vi "220326_STEPN_OCR_v12.vi"(5 "Mode":enum16{"walking", "Repair", "wallet Balance"}(ring), 6 "path to PNG file":path=path "G:/マイドライブ/STEPN_walking/PNG/IMG_5909.PNG" caption="PNG single path") -> (0 "item":string[](array[string])=["Run time", "Step", "Earn GST", "Energy", "Distance", "Date time", "Shoe Lv.", "Shoe #", "durability", "-repair"], 1 "Output String":string[](array[string]), 2 "reading path":path=path "G:/マイドライブ/STEPN_walking/IMG_5909.PNG" caption="PNG single path", 3 "elapsed time(s)":dbl[][](array[numeric]) format="%#_3g", 4 "moji N":i32[](array[numeric]))   [LabVIEW 2016]
uses:
  <vilib>/Utility/file.llb/Write Delimited Spreadsheet (string).vi
  <vilib>/picture/picture.llb/imagedata.ctl
panel:
  out "Boolean":bool
  out "Sumtime(s)":dbl
  in  "File save":bool
  in  "タブ制御器":T1(tab)
  in  "Repair":T2(array[cluster])=[{"left"=300, "top"=529, "right"=508, "bottom"=569}, {"left"=300, "top"=648, "right"=560, "bottom"=677}, {"left"=356, "top"=697, "right"=460, "bottom"=742}]
  in  "walking range":T2(array[cluster])=[{"left"=30, "top"=439, "right"=620, "bottom"=479}, {"left"=430, "top"=668, "right"=620, "bottom"=708}, {"left"=440, "top"=762, "right"=620, "bottom"=802}, {"left"=378, "top"=248, "right"=565, "bottom"=300}, {"left"=123, "top"=296, "right"=350, "bottom"=316}, {"left"=100, "top"=644, "right"=290, "bottom"=664}, {"left"=160, "top"=845, "right"=279, "bottom"=865}, {"left"=150, "top"=891, "right"=242, "bottom"=907}, {"left"=290, "top"=891, "right"=328, "bottom"=907}] caption="walking"
  out "Input picture":picture caption="新規ピクチャ"
  out "image data":T3 caption="画像データ"
  in  "Wallet Balance":T2(array[cluster])=[{"left"=300, "top"=770, "right"=591, "bottom"=830}, {"left"=300, "top"=870, "right"=591, "bottom"=930}, {"left"=300, "top"=970, "right"=591, "bottom"=1030}, {"left"=300, "top"=1070, "right"=591, "bottom"=1130}] caption="wallet Balance"
  out "RANGE":picture
  out "Array":i32[][](array[numeric])
  in  "new flame":T2(array[cluster])=[{"left"=30, "top"=439, "right"=620, "bottom"=479}, {"left"=430, "top"=668, "right"=620, "bottom"=708}, {"left"=440, "top"=762, "right"=620, "bottom"=802}, {"left"=378, "top"=248, "right"=565, "bottom"=300}, {"left"=123, "top"=296, "right"=350, "bottom"=316}, {"left"=100, "top"=644, "right"=290, "bottom"=664}, {"left"=160, "top"=845, "right"=279, "bottom"=865}, {"left"=150, "top"=891, "right"=242, "bottom"=907}, {"left"=290, "top"=891, "right"=328, "bottom"=907}] caption="NEW RANGE"
  in  "RANGE No.":i32
  in  "Range search 2":bool
  out "4-bit pixmap":u8[][][][](array[numeric])
  out "Resized pixmap 2":u8[][][](array[numeric])
  out "string N":i32[](array[numeric])
  in  "new file path (Not A Path if cancelled)":path=path "G:/マイドライブ/STEPN_csv" caption="Save to Path"
  out "Save filename":path
  out "Resized N1 pixmap":i32[][](array[numeric])
  out "N1 Input pic.":picture caption="N1test pic."
  in  "picture No.":i32[](array[numeric])
  out "testdata":T3
  out "identify %":dbl[](array[numeric])
  out "max identify %":dbl
  out "OCR Number":i32
  out "pixcel size (V, Y)":i32[](array[numeric])
  out "Resized (Y, X)":i32[](array[numeric])
  out "Output string":string
  out "Resized N1 pic.":picture caption="Output pic."
  out "Input N1 (Y, X)":i32[](array[numeric])
  out "Ref. pic.":picture caption="fixed pic."
  out "pixcel size(X,Y)":i32[][](array[numeric])
  out "OUtput OCR":string[](array[string])
  out "snipper elapsed time(s) 2":dbl[][][](array[numeric]) format="%.2g"
  out "String":string[](array[string])
  in  "N1_test":bool
  in  "Range search":bool
  out "insert_N":i32[](array[numeric])
  out "max identify % 2":dbl[](array[numeric]) format="%#_3g"
  out "cut picture":picture[](array[picture])
  out "pixel size before":i32[][](array[numeric])
  out "OUtput OCR 2":string[](array[string])
  out "Resized (Y,X)":i32[][](array[numeric])
  out "Resized pic.":picture[](array[picture])
  # "LIST\n0 : runT, STEP (40×30)\n1 : Earn GST (40×30)\n2 : Energy (40×30)\n3 : distance (52×39)\n4 : Date time (20×15)\n5 : shoe Lv. (20×15)\n6 : shoe # (20×15)\n7 : durability (16×12)\n8 : -repair (16×12)"
  # "second"
  # "second"
  # "%"
  # "1"
  # "2"
  # "3"
  # "4"
  # "5"
  # "6"
  # "OFF"
  # "ON"
  # "OFF"
  # "ON"
  # "画像塊"
  # "番号"
  # "OFF"
  # "ON"
  # "c15~¡"
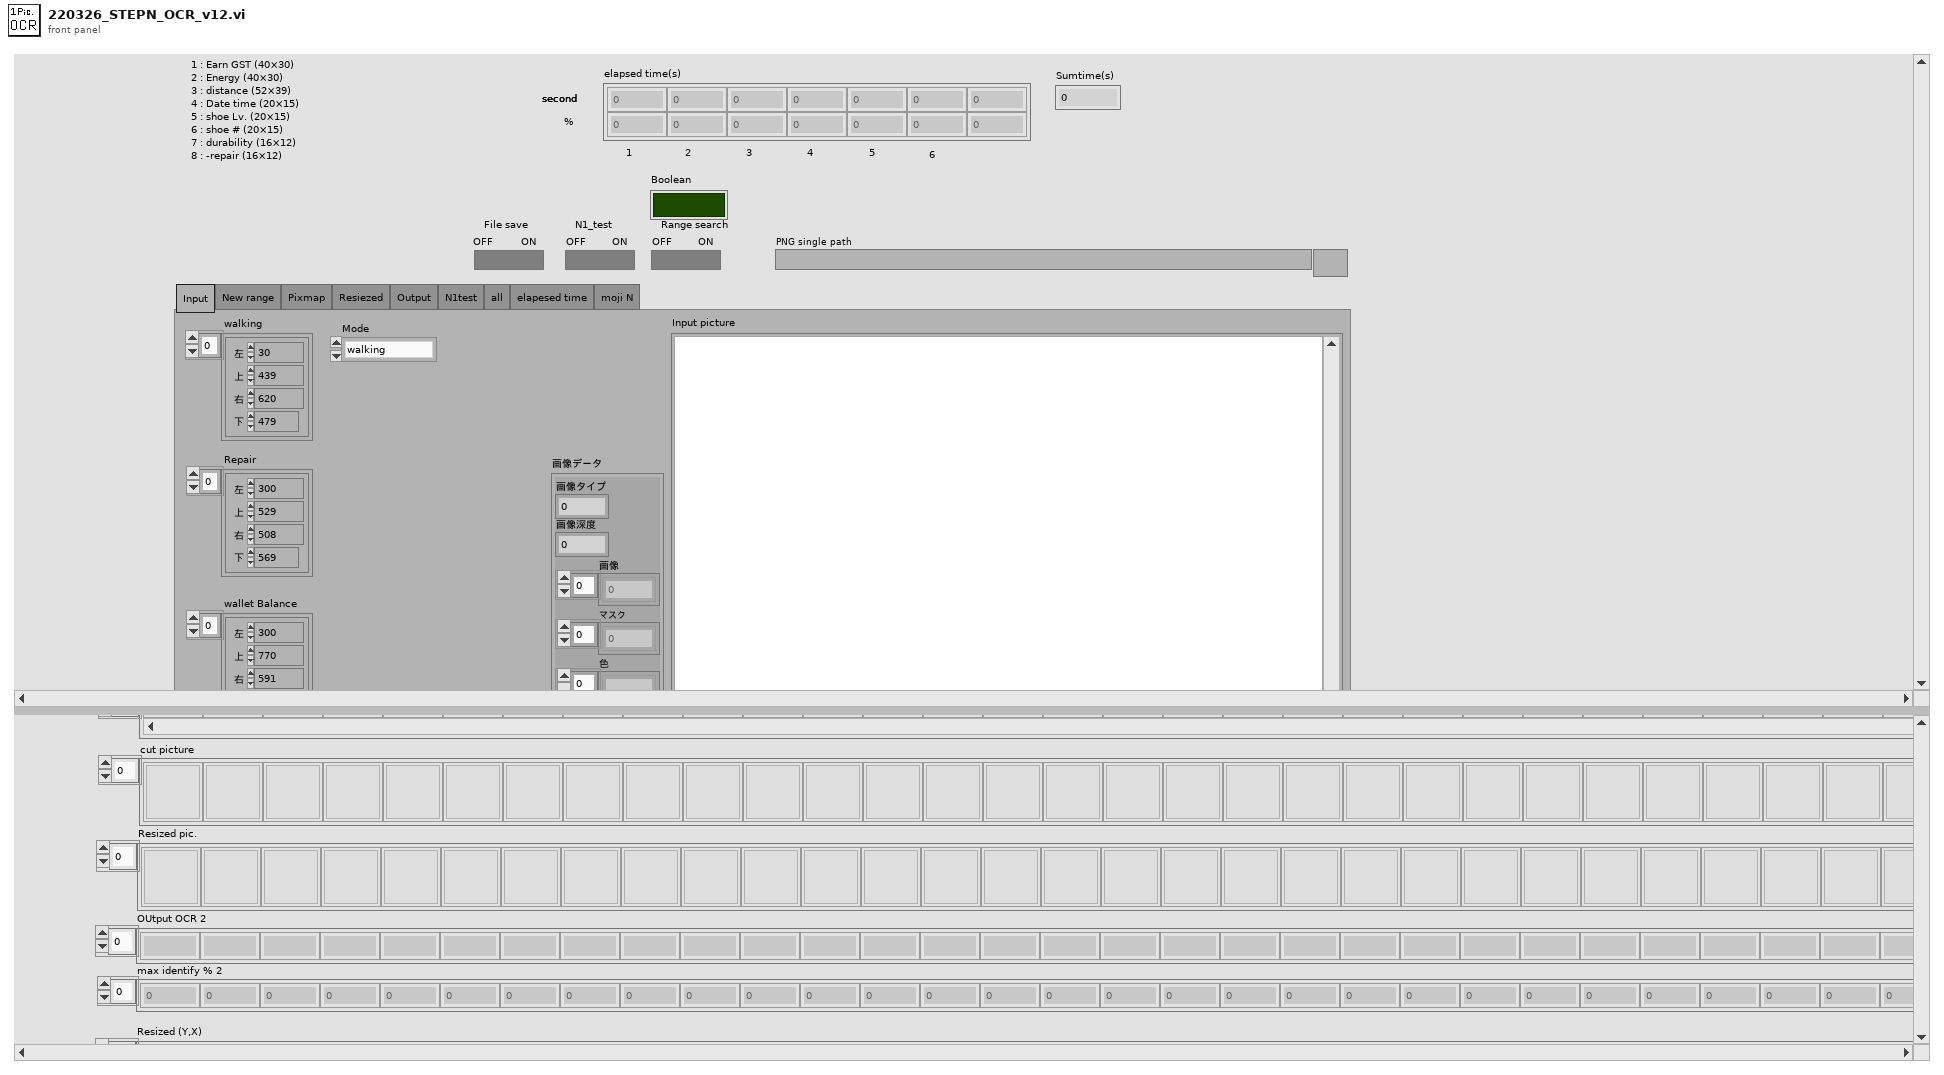
[diagram p1: front panel]
types:
  T1 = enum32{"Input", "New range", "Pixmap", "Resiezed", "Output", "N1test", "all", "elapesed time", "moji N"}
  T2 = cluster{"left":i16, "top":i16, "right":i16, "bottom":i16}[]
  T3 = typedef "imagedata.ctl" = cluster{"image type":i32, "image depth":i32, "image":u8[], "mask":u8[], "colors":u32[], "Rectangle":cluster{"left":i16, "top":i16, "right":i16, "bottom":i16}}
  T4 = cluster{"left":i16, "top":i16, "right":i16, "bottom":i16}
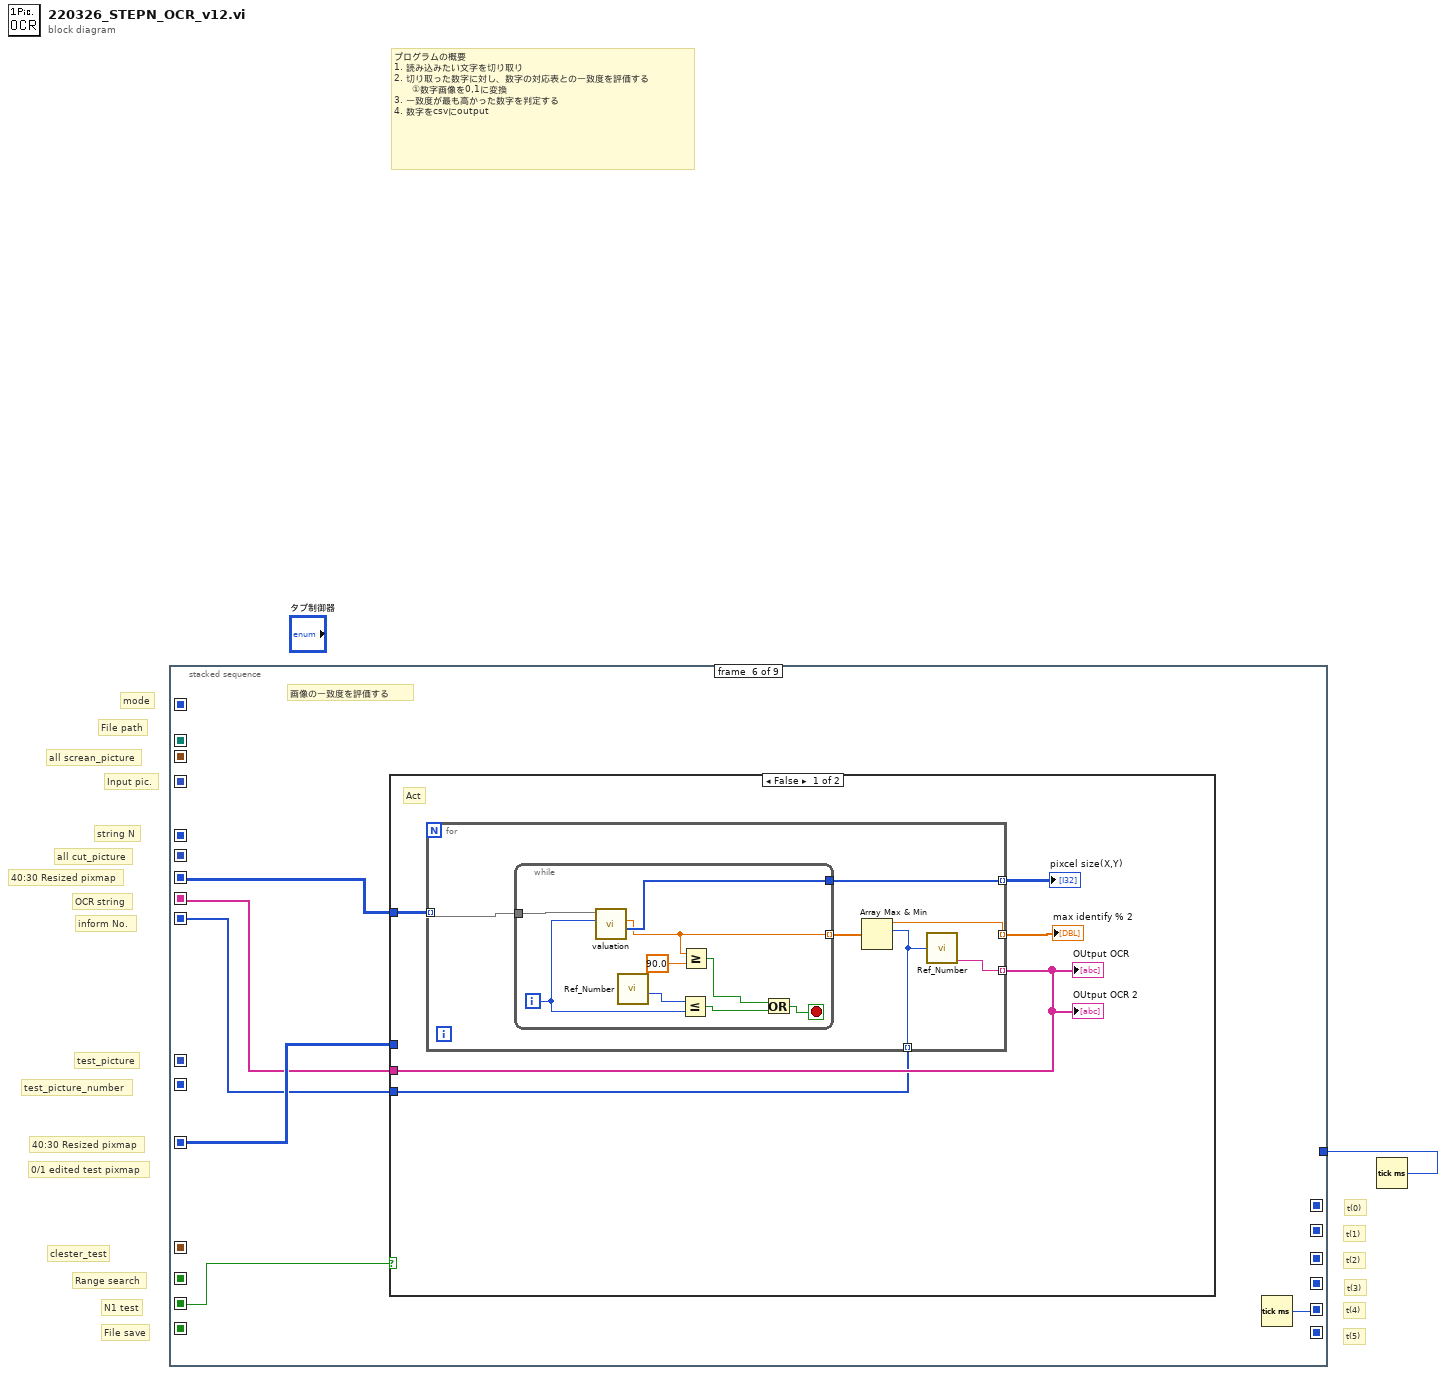
[diagram p0: block diagram]
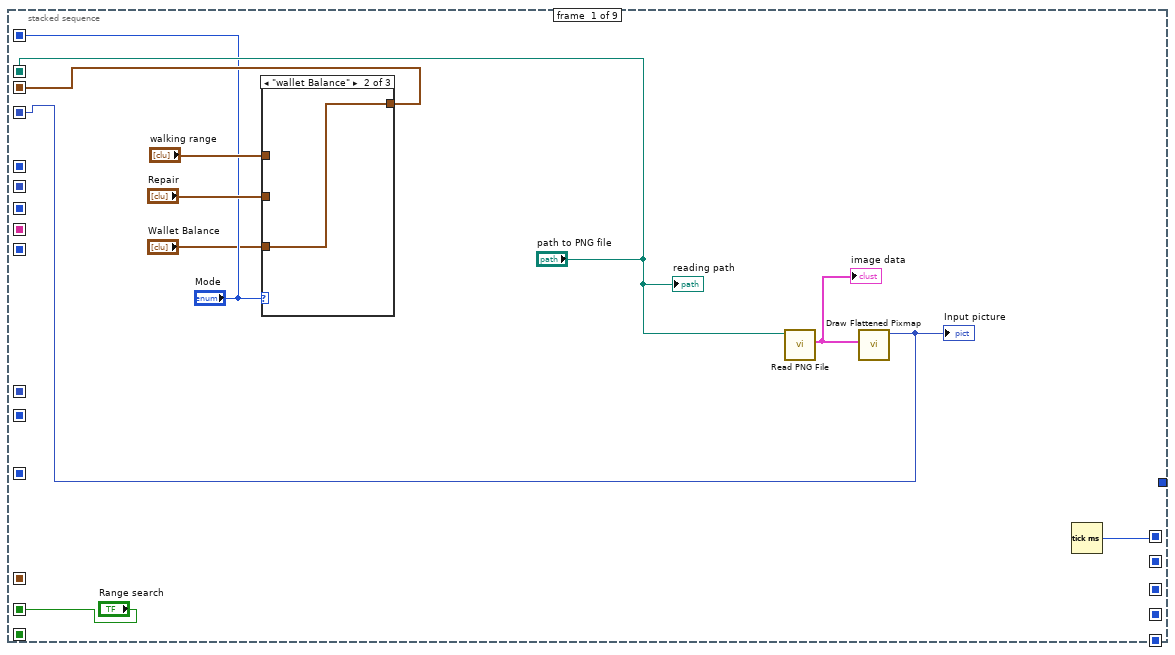
[diagram p2: hidden frame]
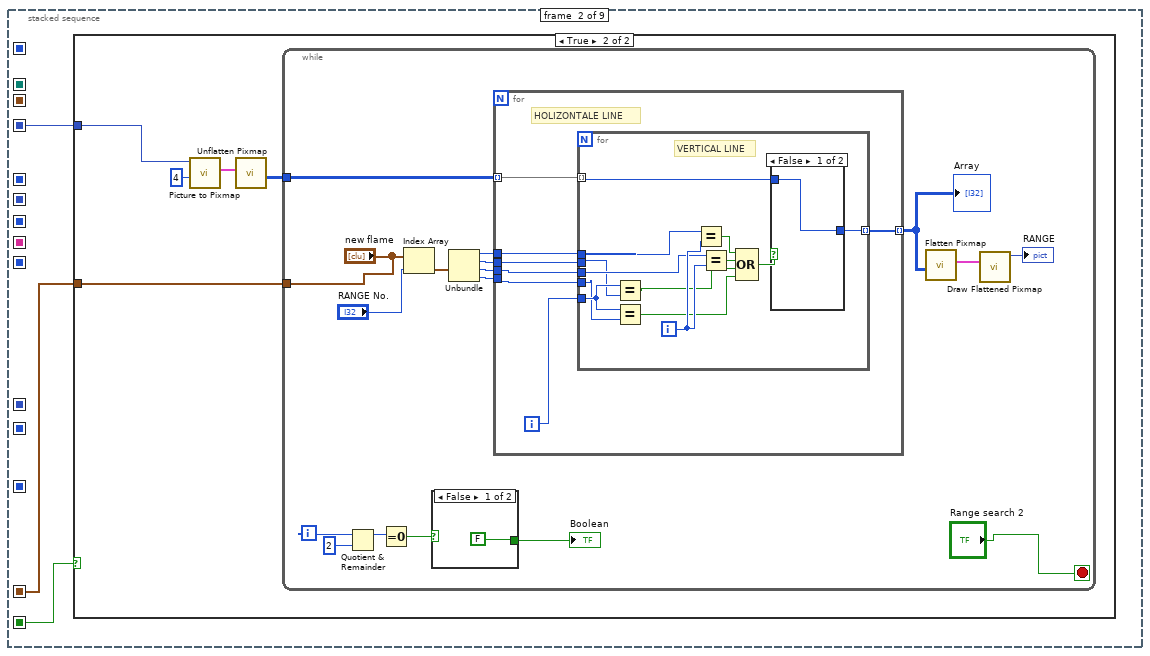
[diagram p5: hidden frame]
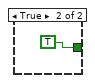
[diagram p7: hidden frame]
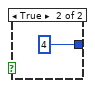
[diagram p8: hidden frame]
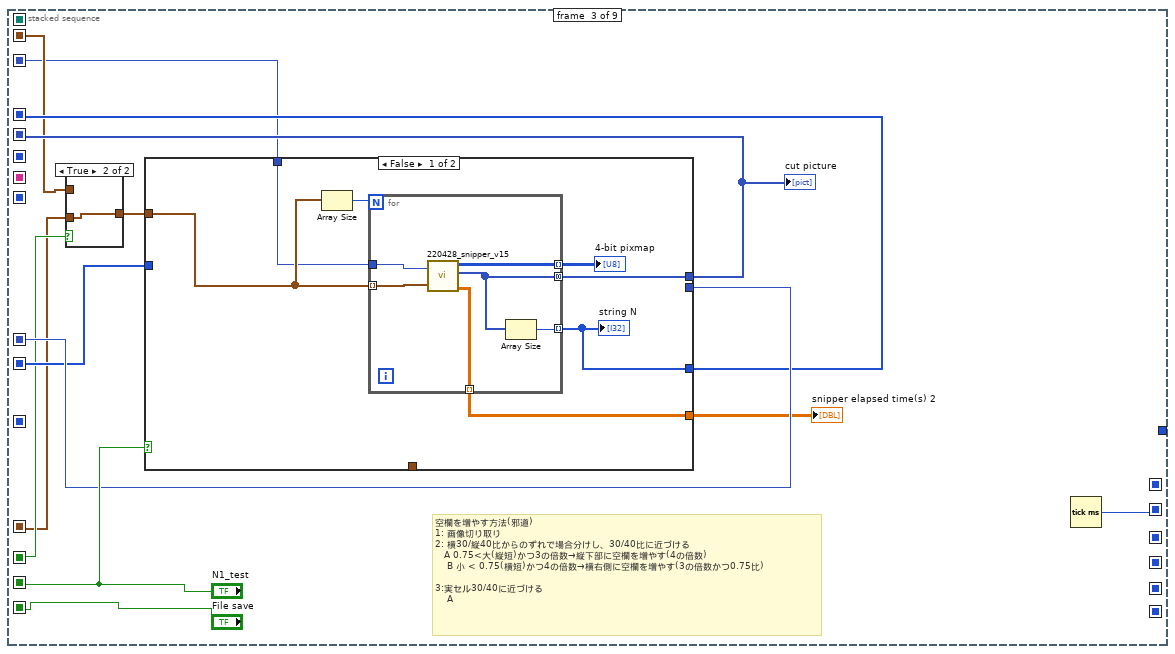
[diagram p9: hidden frame]
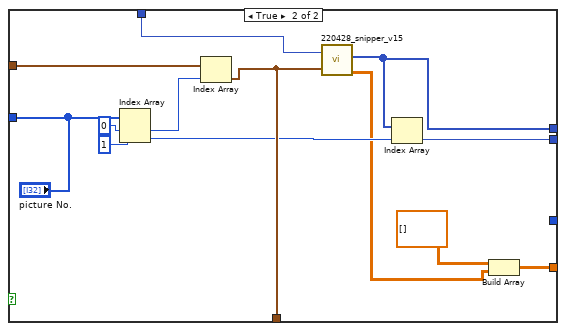
[diagram p11: hidden frame]
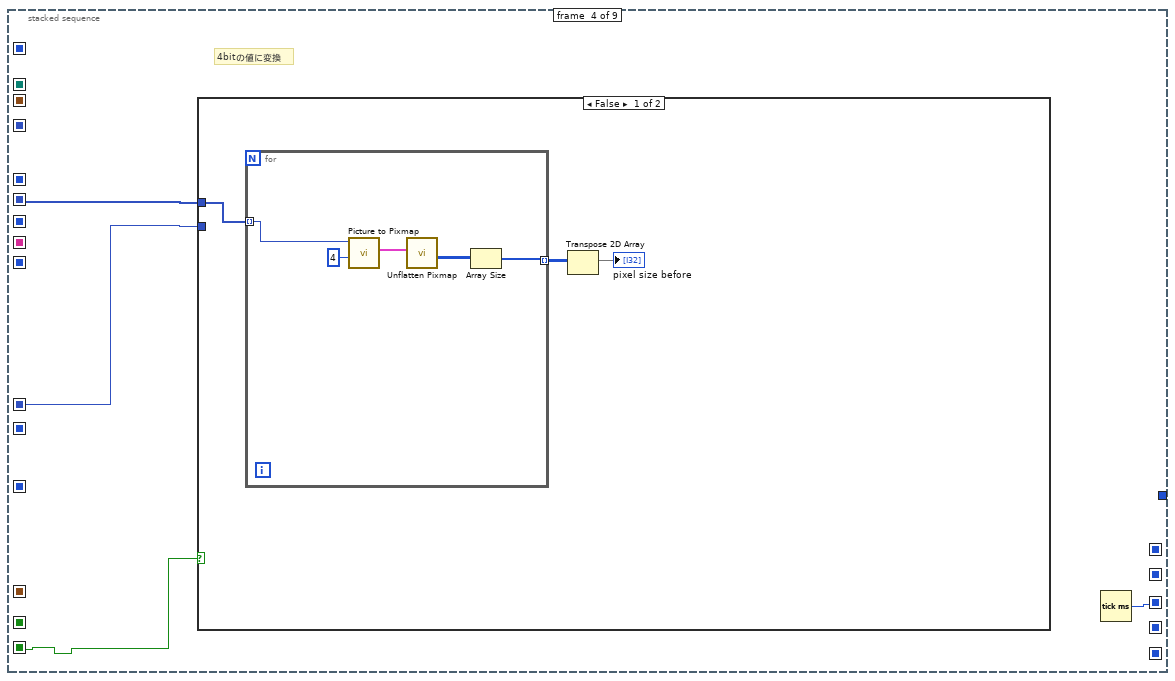
[diagram p12: hidden frame]
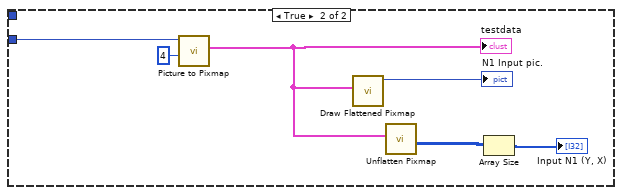
[diagram p13: hidden frame]
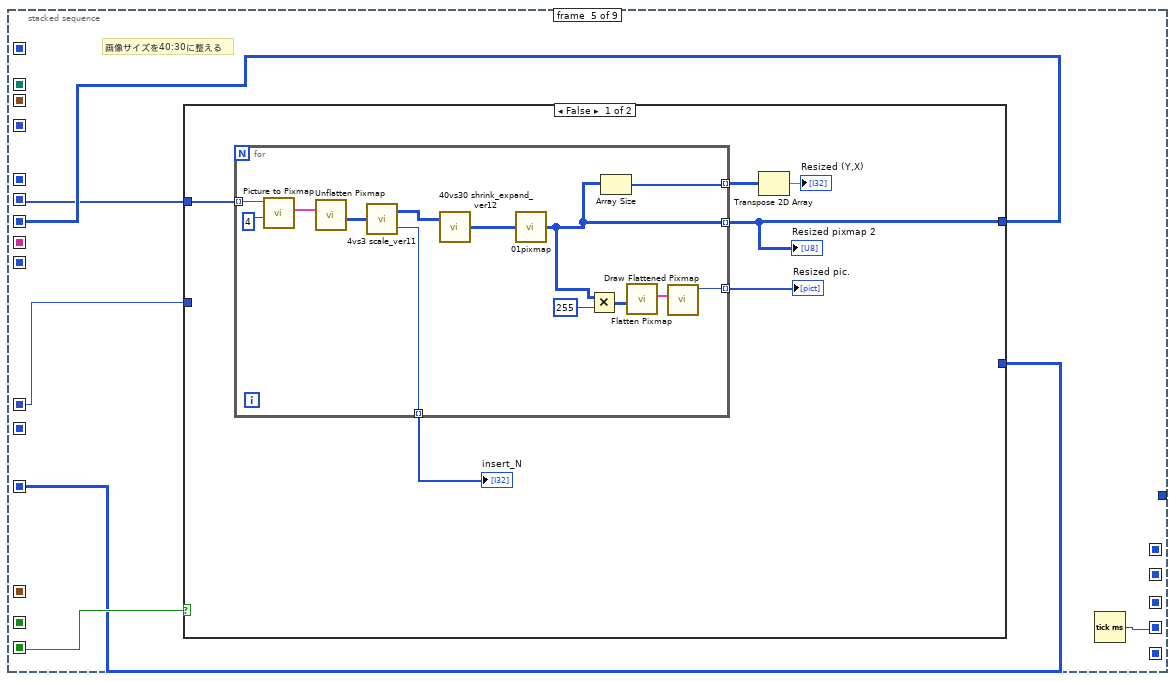
[diagram p14: hidden frame]
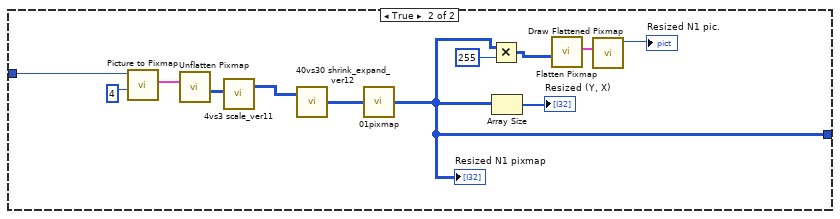
[diagram p15: hidden frame]
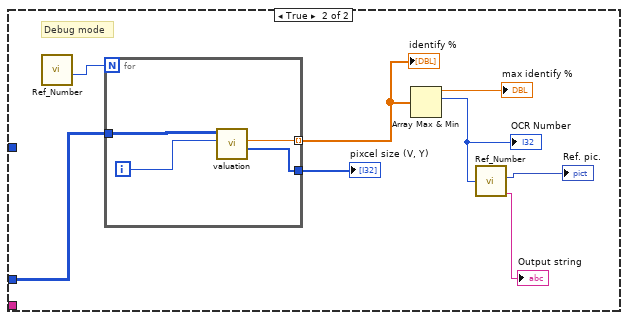
[diagram p16: hidden frame]
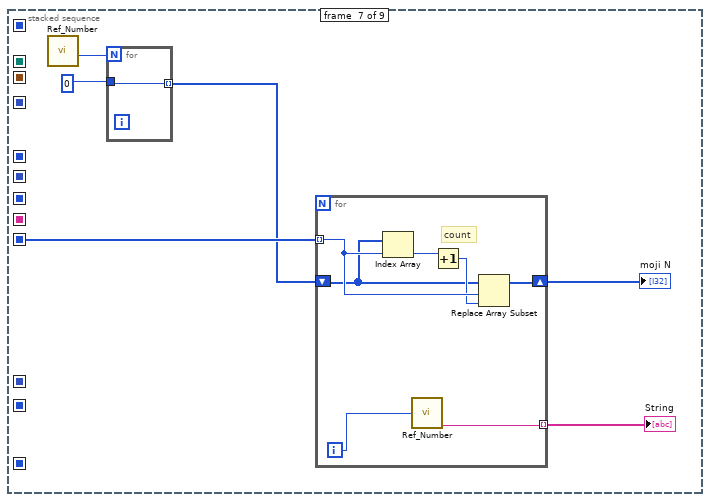
[diagram p17: hidden frame]
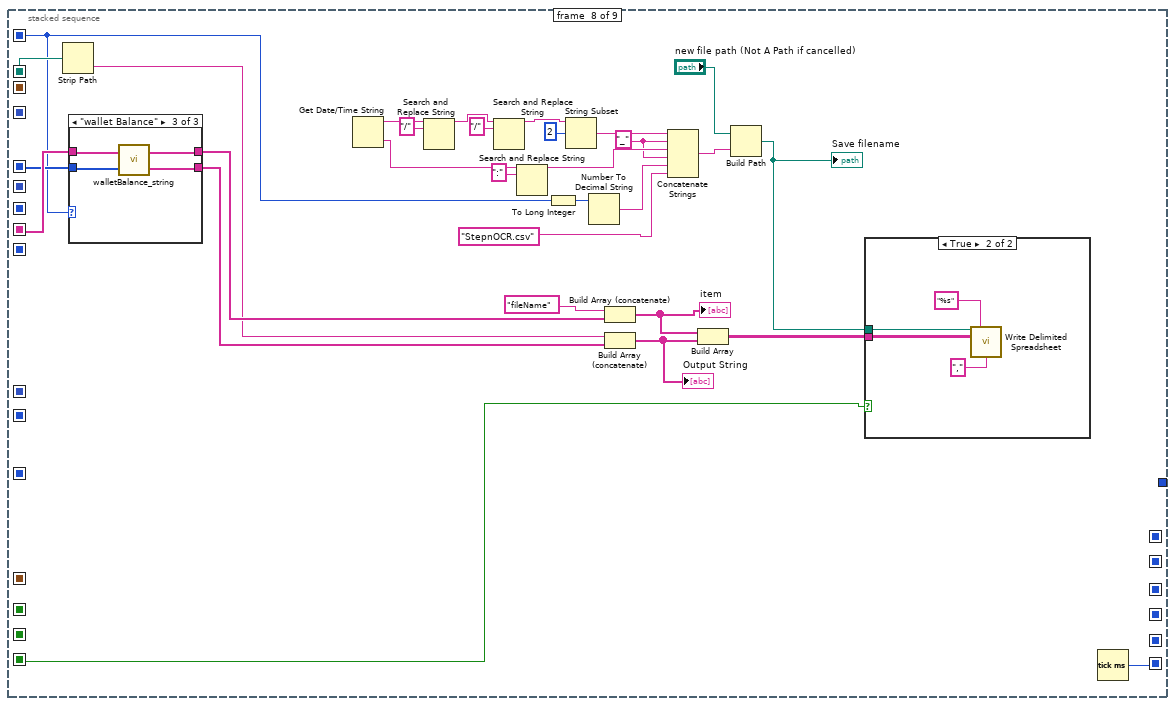
[diagram p18: hidden frame]
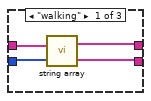
[diagram p19: hidden frame]
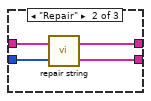
[diagram p20: hidden frame]
diagram:
  # "Input pic."
  # "mode"
  # "inform No."
  # "t(5)"
  # "t(4)"
  # "t(3)"
  # "t(2)"
  # "t(1)"
  # "t(0)"
  # "File save"
  # "string N"
  # "OCR string"
  # "40:30 Resized pixmap"
  # "40:30 Resized pixmap"
  # "0/1 edited test pixmap"
  # "all screan_picture"
  # "all cut_picture"
  # "File path"
  # "clester_test"
  # "test_picture_number"
  # "test_picture"
  # "Range search"
  # "N1 test"
  # "プログラムの概要\n1. 読み込みたい文字を切り取り\n2. 切り取った数字に対し、数字の対応表との一致度を評価する\n　　①数字画像を0,1に変換\n3. 一致度が最も高かった数字を判定する\n4. 数字をcsvにoutput"
  n1 = Tick Count (ms)() -> (millisecond timer value=w1:u32)
  n2 = stacked-sequence {
    seq-local: [_ _ "N1_test" _ _ _ _ _ _] -> [_ _ _ w108 w128 w165 _ _ _]
    seq-local: [_ w16 _ _ _ _ _ _ _] -> [_ _ w65 _ _ _ _ _ _]
    seq-local: ["path to PNG file" _ _ _ _ _ _ _ _] -> [_ _ _ _ _ _ _ w223 _]
    seq-local: [_ _ w75 _ _ _ _ _ _] -> [_ _ _ w106 w124 _ _ _ _]
    seq-local: [_ _ w73 _ _ _ _ _ _] -> [_ _ _ w107 w126 _ _ _ _]
    seq-local: [_ _ w74 _ _ _ _ _ _] -> [_ _ _ _ _ _ _ _ _]
    seq-local: ["Range search" _ _ _ _ _ _ _ _] -> [_ w17 w66 _ _ _ _ _ _]
    seq-local: [_ _ _ _ w125 _ _ _ _] -> [_ _ _ _ _ w163 _ _ _]
    seq-local: [_ _ _ _ w127 _ _ _ _] -> [_ _ _ _ _ w164 _ _ _]
    seq-local: [_ _ _ _ _ w162 _ _ _] -> [_ _ _ _ _ _ _ w241 _]
    seq-local: [_ _ w72 _ _ _ _ _ _] -> [_ _ _ _ _ _ _ w240 _]
    seq-local: [_ _ "File save" _ _ _ _ _ _] -> [_ _ _ _ _ _ _ w224 _]
    seq-local: [w9 _ _ _ _ _ _ _ _] -> [_ _ _ _ _ _ _ _ w269]
    seq-local: [_ _ w70 _ _ _ _ _ _] -> [_ _ _ _ _ _ _ _ w268]
    seq-local: [_ _ _ w105 _ _ _ _ _] -> [_ _ _ _ _ _ _ _ w267]
    seq-local: [_ _ _ _ w123 _ _ _ _] -> [_ _ _ _ _ _ _ _ w266]
    seq-local: [_ _ _ _ _ w161 _ _ _] -> [_ _ _ _ _ _ _ _ w265]
    seq-local: [_ _ _ _ _ _ _ w216 _] -> [_ _ _ _ _ _ _ _ w264]
    seq-local: [_ _ _ _ _ w160 _ _ _] -> [_ _ _ _ _ _ w203 _ _]
    seq-local: [w5 _ _ _ _ _ _ _ _] -> [_ _ w67 _ _ _ _ _ _]
    seq-local: ["Mode" _ _ _ _ _ _ _ _] -> [_ _ _ _ _ _ _ w212 _]
    seq-local: [w2 _ _ _ _ _ _ _ _] -> [_ w15 w64 _ _ _ _ _ _]
    tunnel: w1 -> [_ _ _ _ _ _ _ _ w263]
    frame #0 {
      n3 = case shown="\"wallet Balance\"" "Mode" {
        tunnel: "Repair" -> [w12 _ _]
        tunnel: "walking range" -> [_ _ w14]
        tunnel: [w12 w13 w14] -> w5
        tunnel: "Wallet Balance" -> [_ w13 _]
        frame "Repair" {
        }
        frame "wallet Balance" {
        }
        frame "walking" {
        }
      }
      n4 = call <vilib>:"Read PNG File.vi"("path to PNG file"="path to PNG file") -> ("image data"=w11:T3)  [unwired: 8 in, 2 out]
      "image data" <- w11
      n5 = call <vilib>:"Draw Flattened Pixmap.vi"("image data"=w11) -> ("new picture"=w2:picture)  [unwired: 8 in]
      "Input picture" <- w2
      n6 = Tick Count (ms)() -> (millisecond timer value=w9:u32)
      "reading path" <- "path to PNG file"
    }
    frame #1 {
      n7 = case shown="True" w17 {
        tunnel: [_ w22] -> w16
        tunnel: w15 -> [_ w18]
        frame False {
        }
        frame True {
          n8 = call <vilib>:"Picture to Pixmap.vi"("depth"=4, "picture"=w18) -> ("image data"=w21:T3)  [unwired: 8 in, 1 out]
          n9 = call <vilib>:"Unflatten Pixmap.vi"("image data"=w21) -> ("4-bit pixmap"=w19:u8[][])  [unwired: 4 in, 6 out]
          n10 = while {
            tunnel: w19 -> [w37]
            tunnel: ["new flame"] -> w22
            i -> [w27]
            stop <- "Range search 2" stop-if-true
            n11 = Quotient & Remainder(x=w27, y=2) -> (x-y*floor(x/y)=w25:i32)  [unwired: 1 out]
            n12 = Equal To 0?(x=w25) -> (x = 0?=w24:bool)
            n13 = Index Array(array="new flame", index="RANGE No.") -> (element=w38:T4)
            n14 = case shown="False" w24 {
              tunnel: [FALSE TRUE] -> w23
              frame False {
              }
              frame True {
              }
            }
            "Boolean" <- w23
            n15 = Unbundle(w38) -> ("left"=w31:i16, "top"=w36:i16, "right"=w30:i16, "bottom"=w35:i16)
            n16 = for {
              tunnel: w37 -> [w48] mode=indexing
              tunnel: [w47] -> w34 mode=indexing
              tunnel: w36 -> [w46]
              tunnel: w35 -> [w42]
              tunnel: w31 -> [w45]
              tunnel: w30 -> [w44]
              i -> [w43]
              # "HOLIZONTALE LINE"
              n17 = for {
                tunnel: w48 -> [w58] mode=indexing
                tunnel: [w61] -> w47 mode=indexing
                tunnel: w46 -> [w54]
                tunnel: w45 -> [w57]
                tunnel: w44 -> [w56]
                tunnel: w43 -> [w55]
                tunnel: w42 -> [w53]
                i -> [w59]
                # "VERTICAL LINE"
                n18 = Equal?(x=w55, y=w54) -> (x = y?=w50:bool)
                n19 = Equal?(x=w55, y=w53) -> (x = y?=w49:bool)
                n20 = Equal?(x=w57, y=w59) -> (x = y?=w52:bool)
                n21 = Equal?(x=w56, y=w59) -> (x = y?=w51:bool)
                n22 = Compound Arithmetic op=OR(w52, w51, w50, w49) -> (w60:bool)
                n23 = case shown="False" w60 {
                  tunnel: [w62 4 ("depth")] -> w61
                  tunnel: w58 -> [w62 _]
                  frame False {
                  }
                  frame True {
                  }
                }
              }
            }
            "Array" <- w34
            n24 = call <vilib>:"Flatten Pixmap.vi"("4-bit pixmap"=w34) -> ("image data"=w33:T3)  [unwired: 10 in]
            n25 = call <vilib>:"Draw Flattened Pixmap.vi"("image data"=w33) -> ("new picture"=→"RANGE":picture)  [unwired: 8 in]
          }
        }
      }
    }
    frame #2 {
      # "空欄を増やす方法(邪道)\n1: 画像切り取り\n2: 横30/縦40比からのずれで場合分けし、30/40比に近づける\n   A 0.75<大(縦短)かつ3の倍数→縦下部に空欄を増やす(4の倍数)\n　 B 小 < 0.75(横短)かつ4の倍数→横右側に空欄を増やす(3の倍数かつ0.75比)\n\n3:実セル30/40に近づける\n　 A"
      n26 = case shown="True" w66 {
        tunnel: [w77 w78] -> w68
        tunnel: w67 -> [w77 _]
        tunnel: w65 -> [_ w78]
        frame False {
        }
        frame True {
        }
      }
      n27 = case shown="False" "N1_test" {
        tunnel: [w85 w96] -> w73
        tunnel: [_ w104] -> w75
        tunnel: [_ "picture No."] -> w74
        tunnel: w68 -> [w83 w103]
        tunnel: [_ w98] -> _
        tunnel: [w81 _] -> w72
        tunnel: [w80 w95] -> w69
        tunnel: w64 -> [w79 w92]
        frame False {
          n28 = Array Size(array=w83) -> (size(s)=w84:i32)
          n29 = for {
            N: w84 -> [_]
            tunnel: w79 -> [w91]
            tunnel: w83 -> [w90] mode=indexing
            tunnel: [w88] -> w85 mode=concatenating
            tunnel: [w89] -> w81 mode=indexing
            tunnel: [w87] -> w82 mode=indexing
            tunnel: [w86] -> w80 mode=indexing
            n30 = call "220428_snipper_v15.vi"("Input picture 3"=w91, "hh:mm:ss"=w90) -> ("4-bit pixmap"=w87:u8[][][], "sniped pic."=w88:picture[], "elapsed time(s)"=w86:dbl[][])  [unwired: 1 out]
            n31 = Array Size(array=w88) -> (size(s)=w89:i32)
          }
          "string N" <- w81
          "4-bit pixmap" <- w82
        }
        frame True {
          n32 = Index Array(array="picture No.", index #1=0 ("指標"), index #2=1 ("指標")) -> (element #1=w100:i32, element #2=w97:i32)
          n33 = Index Array(array=w103, index=w100) -> (element=w98:T4)
          n34 = call "220428_snipper_v15.vi"("Input picture 3"=w92, "hh:mm:ss"=w98) -> ("sniped pic."=w96:picture[], "elapsed time(s)"=w93:dbl[][])  [unwired: 2 out]
          n35 = Index Array(array=w96, index=w97) -> (element=w104:picture)
          n36 = Build Array(dbl[][] [], w93) -> (w95:dbl[][][])
        }
      }
      "cut picture" <- w73
      "snipper elapsed time(s) 2" <- w69
      n37 = Tick Count (ms)() -> (millisecond timer value=w70:u32)
    }
    frame #3 {
      # "4bitの値に変換"
      n38 = case shown="False" w108 {
        tunnel: w107 -> [w111 _]
        tunnel: w106 -> [_ w121]
        frame False {
          n39 = for {
            tunnel: w111 -> [w116] mode=indexing
            tunnel: [w113] -> w110 mode=indexing
            n40 = call <vilib>:"Picture to Pixmap.vi"("depth"=4, "picture"=w116) -> ("image data"=w114:T3)  [unwired: 8 in, 1 out]
            n41 = call <vilib>:"Unflatten Pixmap.vi"("image data"=w114) -> ("4-bit pixmap"=w112:u8[][])  [unwired: 4 in, 6 out]
            n42 = Array Size(array=w112) -> (size(s)=w113:i32[])
          }
          n43 = Transpose 2D Array(2D array=w110) -> (transposed array=→"pixel size before":i32[][])
        }
        frame True {
          n44 = call <vilib>:"Picture to Pixmap.vi"("depth"=4, "picture"=w121) -> ("image data"=w119:T3)  [unwired: 8 in, 1 out]
          "testdata" <- w119
          n45 = call <vilib>:"Draw Flattened Pixmap.vi"("image data"=w119) -> ("new picture"=→"N1 Input pic.":picture)  [unwired: 8 in]
          n46 = call <vilib>:"Unflatten Pixmap.vi"("image data"=w119) -> ("4-bit pixmap"=w118:u8[][])  [unwired: 4 in, 6 out]
          n47 = Array Size(array=w118) -> (size(s)=→"Input N1 (Y, X)":i32[])
        }
      }
      n48 = Tick Count (ms)() -> (millisecond timer value=w105:u32)
    }
    frame #4 {
      # "画像サイズを40:30に整える"
      n49 = case shown="False" w128 {
        tunnel: w126 -> [w134 _]
        tunnel: [w132 _] -> w127
        tunnel: [_ w149] -> w125
        tunnel: w124 -> [_ w154]
        frame False {
          n50 = for {
            tunnel: w134 -> [w144] mode=indexing
            tunnel: [w137] -> w132 mode=indexing
            tunnel: [w142] -> w131 mode=indexing
            tunnel: [w140] -> w130 mode=indexing
            tunnel: [w135] -> w129 mode=indexing
            n51 = call <vilib>:"Picture to Pixmap.vi"("depth"=4, "picture"=w144) -> ("image data"=w146:T3)  [unwired: 8 in, 1 out]
            n52 = call <vilib>:"Unflatten Pixmap.vi"("image data"=w146) -> ("4-bit pixmap"=w136:u8[][])  [unwired: 4 in, 6 out]
            n53 = call "4vs3 scale_ver11.vi"("Input bitmap"=w136) -> ("Output bitmap"=w145:i32[][], "insert N"=w135:i32)
            n54 = call "40vs30 shrink_expand_ver12.vi"("Input pic. data"=w145) -> ("Output pixmap"=w143:i32[][])  [unwired: 1 in, 2 out]
            n55 = call "01pixmap.vi"("Input pixmap"=w143) -> ("0/1 pixmap"=w137:i32[][])
            n56 = Multiply(x=w137, y=255) -> (x*y=w138:i32[][])
            n57 = Array Size(array=w137) -> (size(s)=w142:i32[])
            n58 = call <vilib>:"Flatten Pixmap.vi"("4-bit pixmap"=w138) -> ("image data"=w141:T3)  [unwired: 10 in]
            n59 = call <vilib>:"Draw Flattened Pixmap.vi"("image data"=w141) -> ("new picture"=w140:picture)  [unwired: 8 in]
          }
          "Resized pic." <- w130
          "Resized pixmap 2" <- w132
          "insert_N" <- w129
          n60 = Transpose 2D Array(2D array=w131) -> (transposed array=→"Resized (Y,X)":i32[][])
        }
        frame True {
          n61 = call <vilib>:"Picture to Pixmap.vi"("depth"=4, "picture"=w154) -> ("image data"=w158:T3)  [unwired: 8 in, 1 out]
          n62 = call <vilib>:"Unflatten Pixmap.vi"("image data"=w158) -> ("4-bit pixmap"=w157:u8[][])  [unwired: 4 in, 6 out]
          n63 = call "4vs3 scale_ver11.vi"("Input bitmap"=w157) -> ("Output bitmap"=w156:i32[][])  [unwired: 1 out]
          n64 = call "40vs30 shrink_expand_ver12.vi"("Input pic. data"=w156) -> ("Output pixmap"=w151:i32[][])  [unwired: 1 in, 2 out]
          n65 = call "01pixmap.vi"("Input pixmap"=w151) -> ("0/1 pixmap"=w149:i32[][])
          "Resized N1 pixmap" <- w149
          n66 = Multiply(x=w149, y=255) -> (x*y=w148:i32[][])
          n67 = Array Size(array=w149) -> (size(s)=→"Resized (Y, X)":i32[])
          n68 = call <vilib>:"Flatten Pixmap.vi"("4-bit pixmap"=w148) -> ("image data"=w153:T3)  [unwired: 10 in]
          n69 = call <vilib>:"Draw Flattened Pixmap.vi"("image data"=w153) -> ("new picture"=→"Resized N1 pic.":picture)  [unwired: 8 in]
        }
      }
      n70 = Tick Count (ms)() -> (millisecond timer value=w123:u32)
    }
    frame #5 {
      # "画像の一致度を評価する"
      n71 = case shown="False" w165 {
        tunnel: w164 -> [w169 _]
        tunnel: w163 -> [_ w188]
        tunnel: [w167 _] -> w162
        tunnel: [w166 _] -> w160
        frame False {
          # "Act"
          n72 = for {
            tunnel: w169 -> [w175] mode=indexing
            tunnel: [w176] -> w170 mode=indexing
            tunnel: [w173] -> w168 mode=indexing
            tunnel: [w172] -> w167 mode=indexing
            tunnel: [w171] -> w166 mode=indexing
            n73 = while {
              tunnel: w175 -> [w185]
              tunnel: [w184] -> w176
              tunnel: [w181] -> w174 mode=indexing
              i -> [w183]
              stop <- w179 stop-if-true
              n74 = call "valuation.vi"("Input pixmap"=w185, "Ref. N."=w183) -> ("total identify %"=w181:dbl, "vertical × yoko"=w184:i32[])  [unwired: 2 in, 3 out]
              n75 = call "Ref_Number.vi"() -> ("total ref."=w182:i32)  [unwired: 1 in, 3 out]
              n76 = Less Or Equal?(x=w182, y=w183) -> (x <= y?=w178:bool)
              n77 = Greater Or Equal?(x=w181, y=90.0) -> (x >= y?=w177:bool)
              n78 = Or(x=w177, y=w178) -> (x .or. y?=w179:bool)
            }
            n79 = Array Max & Min(array=w174) -> (max value=w173:dbl, max index (indices)=w171:i32)  [unwired: 2 out]
            n80 = call "Ref_Number.vi"("inform N."=w171) -> ("Output string"=w172:string)  [unwired: 3 out]
          }
          "pixcel size(X,Y)" <- w170
          "max identify % 2" <- w168
          "OUtput OCR" <- w167
          "OUtput OCR 2" <- w167
        }
        frame True {
          # "Debug mode"
          n81 = call "Ref_Number.vi"() -> ("total ref."=w190:i32)  [unwired: 1 in, 3 out]
          n82 = for {
            N: w190 -> [_]
            tunnel: w188 -> [w197]
            tunnel: [w196] -> w191
            tunnel: [w195] -> w192 mode=indexing
            i -> [w194]
            n83 = call "valuation.vi"("Input pixmap"=w197, "Ref. N."=w194) -> ("total identify %"=w195:dbl, "vertical × yoko"=w196:i32[])  [unwired: 2 in, 3 out]
          }
          "pixcel size (V, Y)" <- w191
          "identify %" <- w192
          n84 = Array Max & Min(array=w192) -> (max value=→"max identify %":dbl, max index (indices)=w189:i32)  [unwired: 2 out]
          "OCR Number" <- w189
          n85 = call "Ref_Number.vi"("inform N."=w189) -> ("new picture"=→"Ref. pic.":picture, "Output string"=→"Output string":string)  [unwired: 2 out]
        }
      }
      n86 = Tick Count (ms)() -> (millisecond timer value=w161:u32)
    }
    frame #6 {
      n87 = call "Ref_Number.vi"() -> ("total ref."=w202:i32)  [unwired: 1 in, 3 out]
      n88 = for {
        N: w202 -> [_]
        tunnel: 0 -> [w204]
        tunnel: [w204] -> w199 mode=indexing
      }
      n89 = for {
        tunnel: w203 -> [w210] mode=indexing
        shift-right: [w207] -> w201
        shift-left: w199 -> [w208]
        tunnel: [w205] -> w198 mode=indexing
        i -> [w206]
        # "count"
        n90 = Index Array(array=w208, index=w210) -> (element=w211:i32)
        n91 = call "Ref_Number.vi"("inform N."=w206) -> ("Output string"=w205:string)  [unwired: 3 out]
        n92 = Increment(x=w211) -> (x+1=w209:i32)
        n93 = Replace Array Subset(array=w208, new element=w209, index=w210) -> (w207:i32[])
      }
      "moji N" <- w201
      "String" <- w198
    }
    frame #7 {
      w225 = "_" ("文字列")
      n94 = Strip Path(path=w223) -> (name=w220:string)  [unwired: 1 out]
      n95 = case shown="\"wallet Balance\"" w212 {
        tunnel: w241 -> [w244 w249 w253]
        tunnel: w240 -> [w243 w248 w252]
        tunnel: [w242 w247 w251] -> w222
        tunnel: [w245 w246 w250] -> w219
        frame "walking" {
          n96 = call "string array.vi"("String N"=w243, "Input String"=w244) -> ("Output String"=w245:string[], "after item"=w242:string[])
        }
        frame "Repair" {
          n97 = call "repair string.vi"("String N"=w248, "Input String"=w249) -> ("Output String"=w246:string[], "after item 2"=w247:string[])
        }
        frame "wallet Balance" {
          n98 = call "walletBalance_string.vi"("String N"=w252, "Input String"=w253) -> ("Output String"=w250:string[], "after item 2"=w251:string[])
        }
      }
      n99 = Get Date/Time String() -> (date string=w235:string, time string=w231:string)  [unwired: 3 in]
      n100 = Search and Replace String(input string=w235, search string="/" ("検索文字列")) -> (result string=w228:string)  [unwired: 6 in, 3 out]
      n101 = Search and Replace String(input string=w228, search string="/" ("検索文字列")) -> (result string=w227:string)  [unwired: 6 in, 3 out]
      n102 = Search and Replace String(input string=w231, search string=":" ("検索文字列")) -> (result string=w226:string)  [unwired: 6 in, 3 out]
      n103 = To Long Integer(number=w212) -> (32bit integer=w215:i32)
      n104 = String Subset(string=w227, offset (0)=2 ("オフセット（0）")) -> (substring=w230:string)  [unwired: 1 in]
      n105 = Number To Decimal String(number=w215) -> (decimal integer string=w214:string)  [unwired: 1 in]
      n106 = Build Array (concatenate)("fileName", w222) -> (w218:string[])
      "item" <- w218
      n107 = Build Array (concatenate)(w220, w219) -> (w217:string[])
      "Output String" <- w217
      n108 = Concatenate Strings(w230, w225, w226, w225, w214, "StepnOCR.csv") -> (w236:string)
      n109 = Build Array(w218, w217) -> (w239:string[][])
      n110 = Build Path(base path="new file path (Not A Path if cancelled)", name or relative path=w236) -> (appended path=w237:path)
      "Save filename" <- w237
      n111 = case shown="True" w224 {
        tunnel: w239 -> [_ w257]
        tunnel: w237 -> [_ w254]
        frame False {
        }
        frame True {
          n112 = call-poly <vilib>:"Write Delimited Spreadsheet.vi"("file path (dialog if empty)"=w254, "format (%s)"="%s", "2D data"=w257, "delimiter (\\t)"="," ("delimiter (\\t)")) -> ()  [unwired: 10 in, 2 out]
        }
      }
      n113 = Tick Count (ms)() -> (millisecond timer value=w216:u32)
    }
    frame #8 {
      n114 = Build Array(w269, w268, w267, w266, w265, w264) -> (w262:u32[])
      n115 = call "segment time.vi"("Intial time t(0)"=w263, "segment time t(i-1)"=w262) -> ("% time oqupied"=w271:dbl[], "segment time t(i)-t(i-1)"=w270:dbl[])  [unwired: 1 in, 1 out]
      n116 = Build Array(w270, w271) -> (w261:dbl[][])
      "elapsed time(s)" <- w261
      n117 = Index Array(array=w261, index (row)=0 ("指標 （行）")) -> (element=w259:dbl[])  [unwired: 1 in]
      n118 = Add Array Elements(numeric array=w259) -> (sum=→"Sumtime(s)":dbl)
    }
  }
